vi "Create Configured Groups.vi"(8 "error in (no error)":errorcluster, 11 "Task in":refnum<class "Task.lvclass">) -> (0 "error out":errorcluster, 3 "Task out":refnum<class "Task.lvclass">)   [LabVIEW 2020, in "Volatus.lvlib" / "Task.lvclass"]
uses:
  Task.lvclass
  Task.lvclass/Task.ctl
  VolatusConfig/Task/Task.lvclass
  Volatus.lvlib
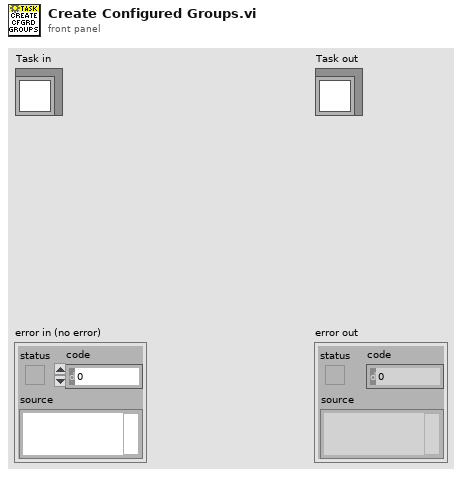
[diagram p1: front panel]
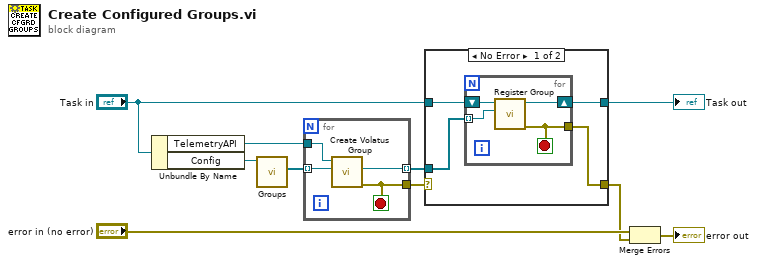
[diagram p0: block diagram]
diagram:
  n1 = Unbundle By Name("Task in") -> ("TelemetryAPI"=w7:refnum<class "TelemetryAPI.lvclass">, "Config"=w9:refnum<class "Task.lvclass">)
  n2 = call "Groups.vi"("Task in"=w9) -> ("Groups"=w8:refnum<class "Group.lvclass">[])  [unwired: 8 in, 2 out]
  n3 = for {
    tunnel: w8 -> [w14] mode=indexing
    tunnel: w7 -> [w13]
    tunnel: [w12] -> w6
    tunnel: [w11] -> w5 mode=indexing
    stop <- w12 stop-if-true
    n4 = call "Create Volatus Group.vi"("Volatus Group"=w14, "TelemetryAPI"=w13) -> ("error out"=w12:errorcluster, "Group"=w11:refnum<class "GroupAbstract.lvclass">)  [unwired: 8 in]
  }
  n5 = case shown="No Error" w6 {
    selector: w6 -> [_ w23]
    tunnel: w5 -> [w17 _]
    tunnel: "Task in" -> [w18 w24]
    tunnel: [w16 w24] -> w3
    tunnel: [w15 w23] -> w1
    frame No Error {
      n6 = for {
        tunnel: w17 -> [w21] mode=indexing
        tunnel: [w19] -> w15
        shift-right: [w20] -> w16
        shift-left: w18 -> [w22]
        stop <- w19 stop-if-true
        n7 = call "Register Group.vi"("Group"=w21, "Task in"=w22) -> ("error out"=w19:errorcluster, "Task out"=w20:refnum<class "Task.lvclass">)  [unwired: 8 in]
      }
    }
    frame Error {
    }
  }
  "Task out" <- w3
  n8 = Merge Errors("error in (no error)", w1) -> (→"error out":errorcluster)
